vi "onStopped.vi"(8 "error in (no error)":errorcluster, 11 "SMO":refnum<class "SMO.lvclass">) -> (0 "error out":errorcluster, 3 "SMO out":refnum<class "SMO.lvclass">)   [LabVIEW 2019, in "SMO.lvclass"]
doc: "JKI State Machine Objects (SMO) 1.3.0.56\nJKI - JKI\nCopyright (c) 2017, JKI"
uses:
  SMO.lvclass
  Typedefs/SMOState --Enum.ctl
  SMO.lvclass/SMO.ctl
  Typedefs/SMO Dependency--Cluster.ctl
  Typedefs/SMO Dependency Event--Cluster.ctl
  Typedefs/SMO Dependency Event--Enum.ctl
  Support/Attribute.Owner/Attribute.Owner.lvclass
panel:
  # "For instructions on how to use the JKI State Machine Objects, examples and video tutorials, visit:\nhttp://jki.net/state-machine-objects/\n\nJKI State Machine Objects™\nhttp://jki.net/state-machine-objects/\nCopyright (C) 2005-2015, JKI <info@jki.net>\nALL RIGHTS RESERVED"
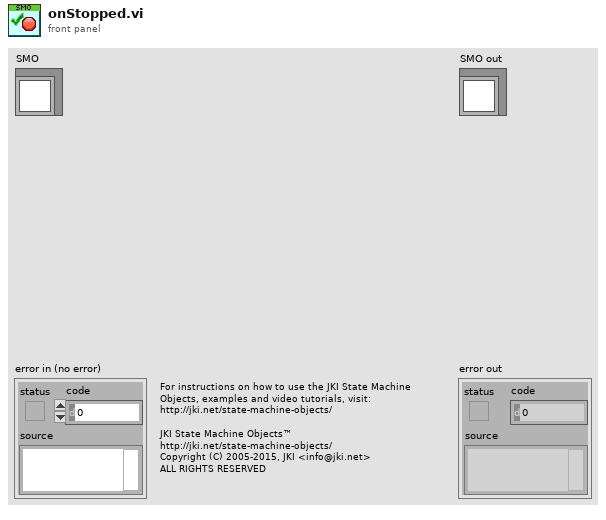
[diagram p1: front panel]
types:
  T1 = typedef "SMO.lvclass/SMOState --Enum.ctl" = enum16{"unknown", "Created", "Started", "Stopped"}
  T2 = typedef "SMO.lvclass/SMO Dependency--Cluster.ctl" = cluster{"Dependency":refnum<class "SMO.lvclass">, "Level":string}
  T3 = typedef "SMO.lvclass/PrivateData--Ref.ctl" = refnum<data-value>
  T4 = typedef "SMO.lvclass/PrivateData--Cluster.ctl" = cluster{"Parent Call":T5, "Registered Processes":T6[], "Sync Notifier":refnum<notifier>, "Process Error Notifier":refnum<notifier>, "Protected Events":T7, "Public Events":T8, "SMO State":T1, "[Dependencies]":T2[], "[Attributes]":refnum<class "Attribute.lvclass">[], "Launcher Close":refnum<notifier>, "Caller Watchdog":refnum<queue>, "Accessibility":T9, "NbStaticDependencies":u32}
  T5 = typedef "SMO.lvclass/Parent Call--Enum.ctl" = enum16{"Allows parent to run", "Does not request parent to run"}
  T6 = typedef "SMO.lvclass/RegisteredProcessData--Cluster.ctl" = cluster{"Name":string, "Static VI Ref":refnum<vi>, "Running":bool, "NotifierRef":u32}
  T7 = typedef "SMO.lvclass/Protected Events.ctl" = cluster{"StopProcesses":refnum<user-event>, "AbortProcesses":refnum<user-event>, "Config Changed":refnum<user-event>, "Dependency":refnum<user-event>}
  T8 = typedef "SMO.lvclass/Public Events.ctl" = cluster{"Error":refnum<user-event>, "State":refnum<user-event>, "Reserve State":refnum<user-event>}
  T9 = typedef "SMO.lvclass/Accessibility--Cluster.ctl" = cluster{"Lock Key":string, "Reserve State":T10}
  T10 = typedef "SMO.lvclass/Reserve State--Enum.ctl" = enum16{"Unreserved", "Reserved", "Self-locked"}
  T11 = typedef "SMO.lvclass/SMO Dependency Event--Cluster.ctl" = cluster{"Name":string, "GUID":string, "Event":T12}
  T12 = typedef "SMO.lvclass/SMO Dependency Event--Enum.ctl" = enum16{"Added", "Removed", "Started", "Stopped"}
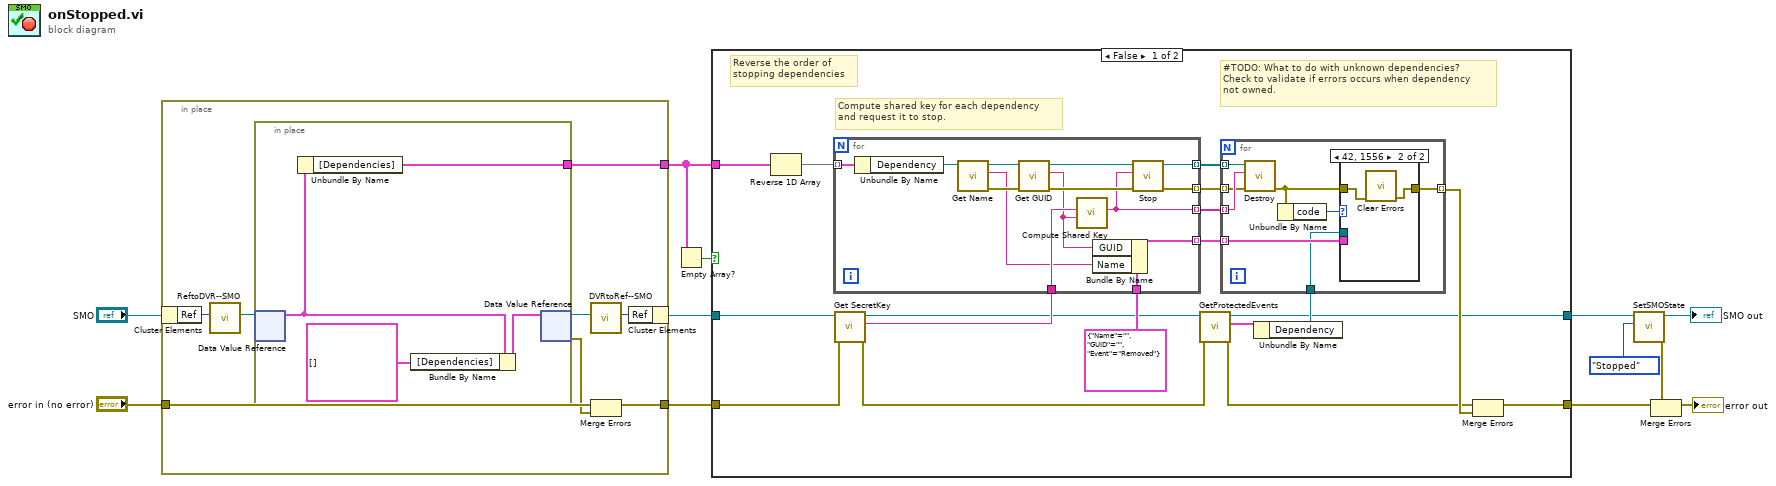
[diagram p0: block diagram]
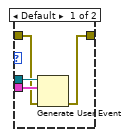
[diagram p2: hidden frame]
diagram:
  n1 = in-place {
    in-place-border: "error in (no error)" -> [w16]
    in-place-border: [w14] -> w3
    in-place-border: [w13] -> w1
    n2 = in-place-cluster #1("SMO") -> ("Ref"=w20:u32)
    n3 = call "ReftoDVR--SMO.vi"("Ref"=w20) -> ("Ref"=w19:T3)  [unwired: 10 in]
    n4 = in-place {
      in-place-border: [w24] -> w13
      n5 = in-place-dvr #2(w19) -> (w23:T4)  [unwired: 1 out]
      n6 = Unbundle By Name(w23) -> ("[Dependencies]"=w24:T2[])
      n7 = Bundle By Name(cluster=w23, "[Dependencies]"=T2[] []) -> (w22:T4)
      n8 = in-place-dvr #2(w22) -> (w18:T3, w15:errorcluster)
    }
    n9 = call "DVRtoRef--SMO.vi"("Ref"=w18) -> ("Ref"=w17:u32)  [unwired: 10 in]
    n10 = Merge Errors(w16, w15) -> (w14:errorcluster)
    n11 = in-place-cluster #1("Ref"=w17) -> (w4:refnum<class "SMO.lvclass">)
  }
  n12 = Empty Array?(array=w1) -> (empty?=w2:bool)
  n13 = case shown="False" w2 {
    tunnel: [w42 w71] -> w5
    tunnel: w1 -> [w41 _]
    tunnel: w4 -> [w40 w72]
    tunnel: w3 -> [w39 w71]
    tunnel: [w25 w72] -> w7
    frame False {
      # "#TODO: What to do with unknown dependencies?\nCheck to validate if errors occurs when dependency\nnot owned."
      # "Reverse the order of\nstopping dependencies"
      # "Compute shared key for each dependency\nand request it to stop."
      n14 = Reverse 1D Array(array=w41) -> (reversed array=w37:T2[])
      n15 = call "Get SecretKey.vi"("error in (no error)"=w39, "SMO"=w40) -> ("error out"=w29:errorcluster, "SecretKey"=w38:string, "SMO out"=w30:refnum<class "SMO.lvclass">)  [unwired: 7 in]
      n16 = for {
        tunnel: w37 -> [w67] mode=indexing
        tunnel: w38 -> [w69]
        tunnel: [w66] -> w36 mode=indexing
        tunnel: [w65] -> w35 mode=indexing
        tunnel: [w64] -> w34 mode=indexing
        tunnel: T11 {"Name"="", "GUID"="", "Event"=enum."Removed"} ("Dependency Event") -> [w58]
        tunnel: [w57] -> w31 mode=indexing
        n17 = Unbundle By Name(w67) -> ("Dependency"=w63:refnum<class "SMO.lvclass">)
        n18 = call "Get Name.vi"("SMO"=w63) -> ("error out"=w61:errorcluster, "Name"=w59:string, "SMO out"=w62:refnum<class "SMO.lvclass">)  [unwired: 8 in]
        n19 = call "Get GUID.vi"("error in (no error)"=w61, "SMO"=w62) -> ("error out"=w68:errorcluster, "GUID"=w60:string, "SMO out"=w70:refnum<class "SMO.lvclass">)  [unwired: 7 in]
        n20 = call "Compute Shared Key.vi"("GUID"=w60, "SecretKey"=w69) -> ("Shared Key"=w65:string)  [unwired: 9 in]
        n21 = Bundle By Name(cluster=w58, "GUID"=w60, "Name"=w59) -> (w57:T11)
        n22 = call "Stop.vi"("error in (no error)"=w68, "Shared Key"=w65, "SMO"=w70) -> ("error out"=w64:errorcluster, "SMO out"=w66:refnum<class "SMO.lvclass">)  [unwired: 7 in]
      }
      n23 = call "GetProtectedEvents.vi"("error in (no error)"=w29, "SMO"=w30) -> ("error out"=w28:errorcluster, "SMO Protected Events"=w27:T7, "SMO out"=w25:refnum<class "SMO.lvclass">)  [unwired: 7 in]
      n24 = Unbundle By Name(w27) -> ("Dependency"=w26:refnum<user-event>)
      n25 = for {
        tunnel: w36 -> [w50] mode=indexing
        tunnel: w35 -> [w49] mode=indexing
        tunnel: [w45] -> w33 mode=indexing
        tunnel: w34 -> [w48] mode=indexing
        tunnel: w31 -> [w44] mode=indexing
        tunnel: w26 -> [w43]
        n26 = call "Destroy.vi"("error in (no error)"=w48, "Shared Key"=w49, "SMO"=w50) -> ("error out"=w46:errorcluster)  [unwired: 8 in]
        n27 = Unbundle By Name(w46) -> ("code"=w47:i32)
        n28 = case shown="42, 1556" w47 {
          tunnel: w46 -> [w52 w56]
          tunnel: [w51 w55] -> w45
          tunnel: w44 -> [w53 _]
          tunnel: w43 -> [w54 _]
          frame Default {
            n29 = Generate User Event(user event=w54, event data cluster=w53, error in=w52) -> (error out=w51:errorcluster)  [unwired: 1 in, 1 out]
          }
          frame 42, 1556 {
            n30 = call <vilib>:"Clear Errors.vi"("error in (no error)"=w56) -> ("error out"=w55:errorcluster)  [unwired: 5 in, 1 out]
          }
        }
      }
      n31 = Merge Errors(w28, w33) -> (w42:errorcluster)
    }
    frame True {
    }
  }
  n32 = call "SetSMOState.vi"("SMO State"=SMOState_--Enum."Stopped" ("event data"), "SMO in"=w7) -> ("error out"=w11:errorcluster, "SMO out"=→"SMO out":refnum<class "SMO.lvclass">)  [unwired: 8 in]
  n33 = Merge Errors(w5, w11) -> (→"error out":errorcluster)
